vi "string parse mathematica list assosiated array -- V2.vi"(6 "pattern":string="^[\\t \\r \\n \\s \\, ]*\\\"(.+?)\\\"[\\t \\r \\n \\s]*\\-\\>[\\t \\r \\n \\s]*\\<\\|([^\\|]+)\\|\\>", 7 "action":T2=enum."parse string", 8 "array of inds":dbl[](array[numeric]), 9 "array of IDs":string[](array[string]), 10 "Map IN":map{string, map{T1, dbl}}(c390), 11 "string IN":string="\"014_042324\" ->   <|  \n\"T\"->  0.50  , \n\"θ\"-> 50 , \n\"vproj\" ->  0.3,\n\"B\" -> 60 ,\n\"plain\" -> \"bc\"\n  |>   , \n  \n\"012_042324\" ->   <|  \n\"T\"->  0.50  , \n\"θ\"-> 70  , \n\"vproj\" -> 0.5,\n\"plain\" -> \"bc\"\n  |>   ,  \n  \n  \n  ") -> (0 "items actually found":T1[](array[typedef])=[enum."T (K)", enum."B (T)", enum."θ (deg)"], 1 "actually found Map OUT":map{string, map{T1, dbl}}(c390)={"012_042324"={enum."T (K)"=0.5, enum."B (T)"=0.0, enum."θ (deg)"=70.0}, "014_042324"={enum."T (K)"=0.5, enum."B (T)"=60.0, enum."θ (deg)"=50.0}}, 2 "all keys Map OUT":map{string, map{T1, dbl}}(c390)={"012_042324"={enum."ζ"=0.0, enum."τ1"=0.0, enum."τS"=0.0, enum."τN"=0.0, enum."τC"=0.0, enum."κ0"=0.0, enum."m1"=0.0, enum."m2"=0.0, enum."m3"=0.0, enum."T (K)"=0.5, enum."B (T)"=0.0, enum."θ (deg)"=70.0, enum."Re(offset)"=0.0, enum."Im(offset)"=0.0, enum."στ1"=0.0, enum."στS"=0.0, enum."στN"=0.0, enum."τ11"=0.0, enum."τ12"=0.0, enum."τ22"=0.0, enum."τN1"=0.0, enum."τN2"=0.0, enum."σηlogτ1"=0.0, enum."σηlogτS"=0.0, enum."σηlogτN"=0.0, enum."σlogτ1"=0.0, enum."σlogτS"=0.0, enum."σlogτN"=0.0, enum."σητ1"=0.0, enum."σητS"=0.0, enum."σητN"=0.0, enum."noiseT"=0.0, enum."plain"=0.0, enum."vproj"=0.0}, "014_042324"={enum."ζ"=0.0, enum."τ1"=0.0, enum."τS"=0.0, enum."τN"=0.0, enum."τC"=0.0, enum."κ0"=0.0, enum."m1"=0.0, enum."m2"=0.0, enum."m3"=0.0, enum."T (K)"=0.5, enum."B (T)"=60.0, enum."θ (deg)"=50.0, enum."Re(offset)"=0.0, enum."Im(offset)"=0.0, enum."στ1"=0.0, enum."στS"=0.0, enum."στN"=0.0, enum."τ11"=0.0, enum."τ12"=0.0, enum."τ22"=0.0, enum."τN1"=0.0, enum."τN2"=0.0, enum."σηlogτ1"=0.0, enum."σηlogτS"=0.0, enum."σηlogτN"=0.0, enum."σlogτ1"=0.0, enum."σlogτS"=0.0, enum."σlogτN"=0.0, enum."σητ1"=0.0, enum."σητS"=0.0, enum."σητN"=0.0, enum."noiseT"=0.0, enum."plain"=0.0, enum."vproj"=0.0}}, 3 "string out":string="\"014_042324\" ->   <|  \n\"T\"->  0.50  , \n\"θ\"-> 50 , \n\"vproj\" = 0.3,\n\"B\" -> 60 ,\n\"plain\" -> \"bc\"\n  |>   , \n  \n\"012_042324\" ->   <|  \n\"T\"->  0.50  , \n\"θ\"-> 70  , \n\"vproj\" = 0.5,\n\"plain\" -> \"bc\"\n  |>   ,  \n  \n  \n  ")   [LabVIEW 2021]
uses:
  3-lorentzian-heat-response action.ctl
  3-lorentzian-parameters.ctl
  mathematica string map action.ctl
  3-lorentzian-heat-response -- V4.vi/142dd4c5-f9ed-c64b-bc14-a88e3e2c450a.vi
  <vilib>/Analysis/polynomials.llb/Polynomial Roots.vi
  <vilib>/Analysis/polynomials.llb/Polynomial Roots (DBL).vi
  <vilib>/Comparison/Less/Less Functor/Less Functor.lvclass
  <vilib>/regexp/Match Regular Expression.xnode
panel:
  out "after match":string
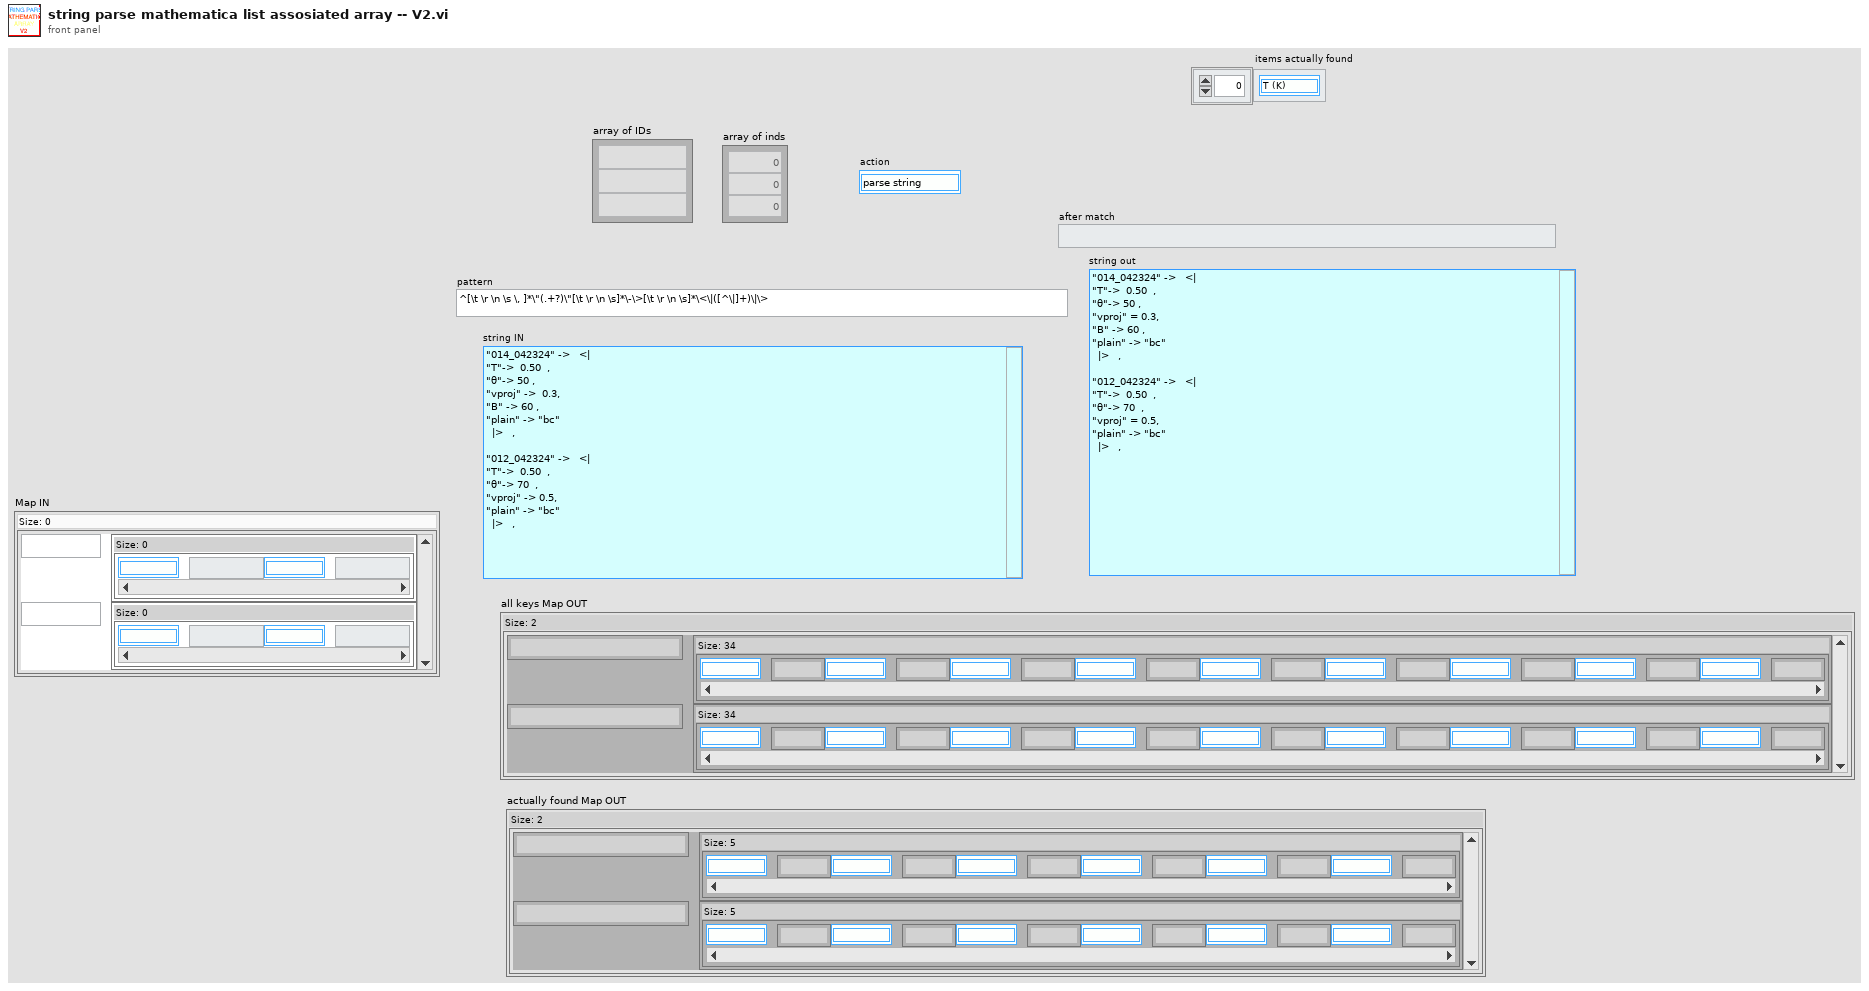
[diagram p1: front panel]
types:
  T1 = typedef "3-lorentzian-parameters.ctl" = enum16{"ζ", "τ1", "τS", "τN", "τC", "κ0", "m1", "m2", "m3", "T (K)", "B (T)", "θ (deg)", "side (S|R)", "set of (B|T)", "Re(offset)", "Im(offset)", "στ1", "στ1-", "στ1+", "στS", "στS-", "στS+", "στN", "στN-", "στN+", "τ11", "τ12", "τ21", "τ22", "τN1", "τN2", "σηlogτ1", "σηlogτS", "σηlogτN", "σlogτ1", "σlogτS", "σlogτN", "σητ1", "σητS", "σητN", "noiseT", "plain", "vproj"}
  T2 = typedef "3-lorentzian-heat-response action.ctl" = enum16{"calc R", "create string", "calc m1m2m3", "dζ", "dT1", "dτS", "dτN", "dτC", "d-all", "dκ0", "T(K)", "m1", "m2", "m3", "parse string", "θ (deg)", "B (T)", "onlygrads", "newton", "create emty string", "simple2nd", "calc R2", "ScalarProd", "ScalarProd-diff", "nothing", "ScalarProd-eta", "tolog", "ignore", "three2nd", "eta-errors"}
  T3 = typedef "mathematica string map action.ctl" = enum16{"create string", "calc m1m2m3", "parse string"}
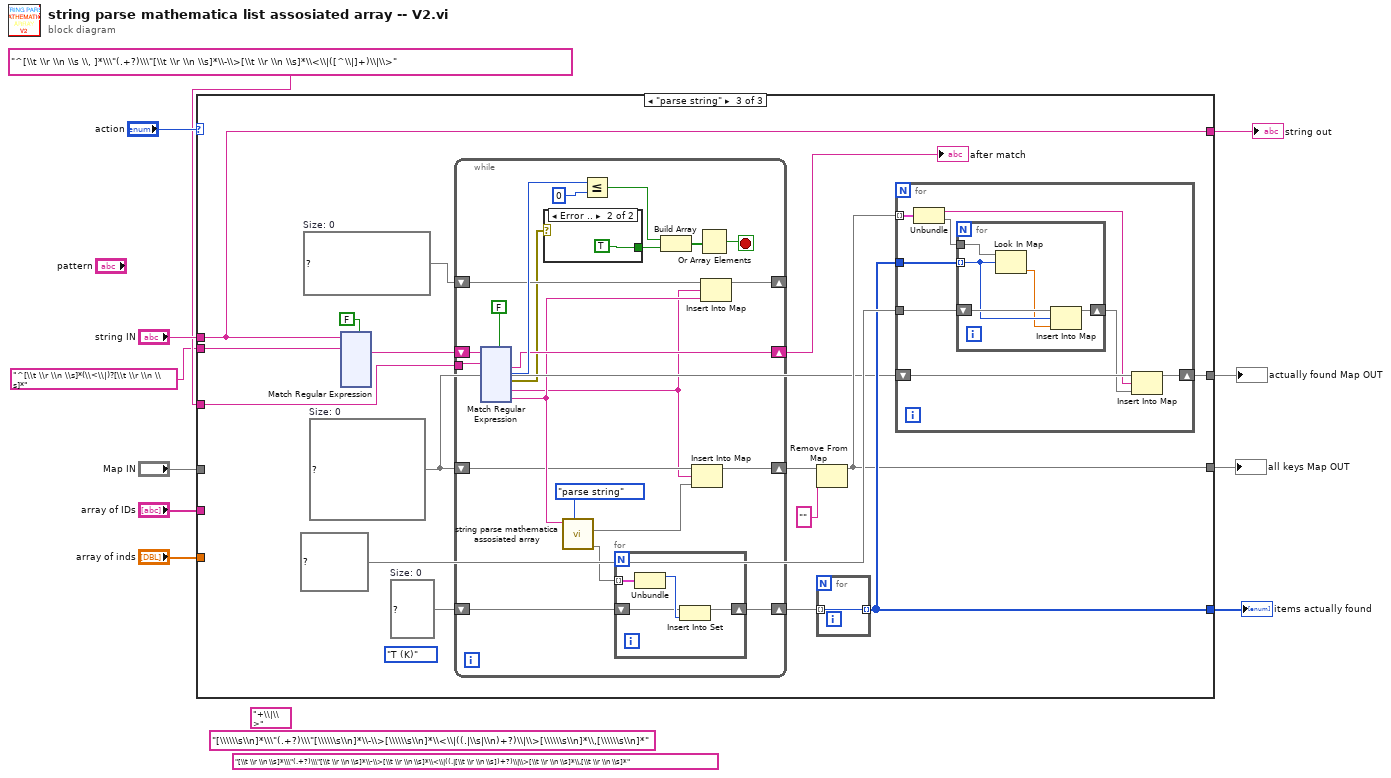
[diagram p0: block diagram]
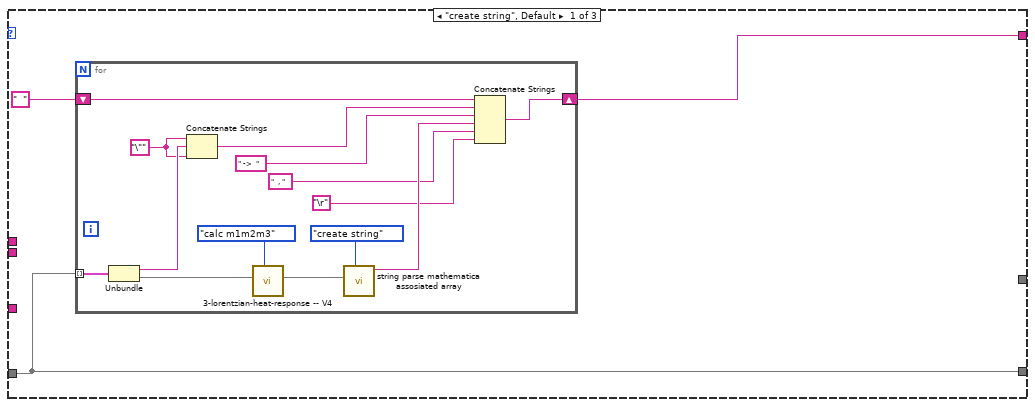
[diagram p2: hidden frame]
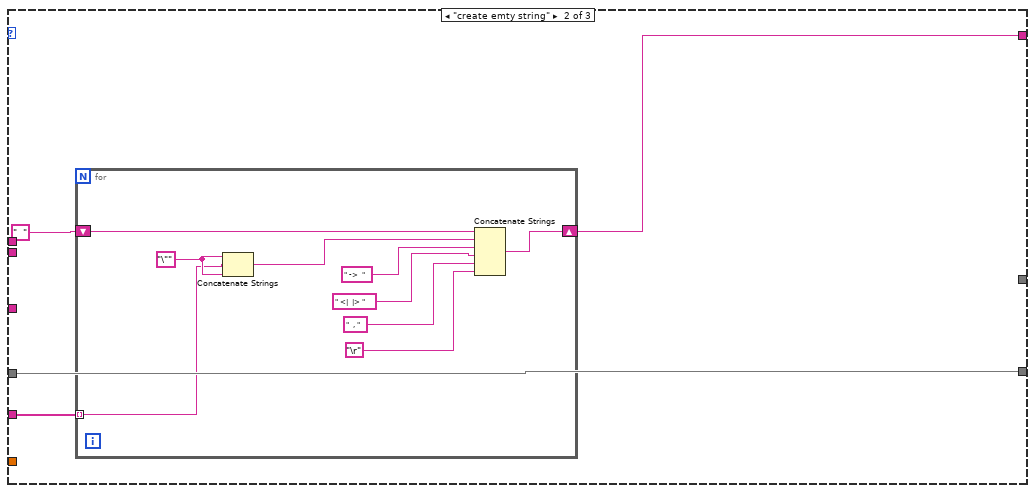
[diagram p3: hidden frame]
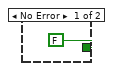
[diagram p4: hidden frame]
diagram:
  (unwired) "+\\|\\>" ("format string")
  (unwired) "[\\t \\r \\n \\s]*\\\"(.+?)\\\"[\\t \\r \\n \\s]*\\-\\>[\\t \\r \\n \\s]*\\<\\|((.|[\\t \\r \\n \\s])+?)\\|\\>[\\t \\r \\n \\s]*\\,[\\t \\r \\n \\s]*" ("pattern")
  (unwired) "[\\\\\\s\\n]*\\\"(.+?)\\\"[\\\\\\s\\n]*\\-\\>[\\\\\\s\\n]*\\<\\|((.|\\s|\\n)+?)\\|\\>[\\\\\\s\\n]*\\,[\\\\\\s\\n]*" ("pattern")
  n1 = case shown="\"parse string\"" "action" {
    tunnel: "string IN" -> [_ _ w53]
    tunnel: [w12 w30 w45] -> w6
    tunnel: "Map IN" -> [w12 w30 _]
    tunnel: [w14 w32 w53] -> w8
    tunnel: "array of inds" -> [_ _ _]
    tunnel: "array of IDs" -> [_ w29 _]
    tunnel: "^[\\t \\r \\n \\s \\, ]*\\\"(.+?)\\\"[\\t \\r \\n \\s]*\\-\\>[\\t \\r \\n \\s]*\\<\\|([^\\|]+)\\|\\>" ("pattern") -> [_ _ w49]
    tunnel: [_ _ w46] -> w3
    tunnel: [_ _ w44] -> w2
    tunnel: "^[\\t \\r \\n \\s]*(\\<\\|)?[\\t \\r \\n \\s]*" ("format string") -> [_ _ w42]
    frame "create string", Default {
      n2 = for {
        tunnel: w12 -> [w28] mode=indexing
        shift-right: [w22] -> w14
        shift-left: "  " ("all string") -> [w23]
        w15 = "\"" ("all string")
        n3 = Unbundle(w28) -> ("after match 3"=w17:string, "Map"=w20:map{T1, dbl})
        n4 = Concatenate Strings(w15, w17, w15) -> (w16:string)
        n5 = call "3-lorentzian-heat-response -- V4.vi"("action"=3-lorentzian-heat-response_action."calc m1m2m3", "Map IN"=w20) -> ("Map OUT"=w18:map{T1, dbl})  [unwired: 7 in, 2 out]
        n6 = call "string parse mathematica assosiated array.vi"("action"=mathematica_string_map_action."create string" ("derivative"), "map IN"=w18) -> ("String OUT"=w26:string)  [unwired: 7 in, 2 out]
        n7 = Concatenate Strings(w23, w16, " ->  " ("all string"), w26, "  , " ("all string"), "\r") -> (w22:string)
      }
    }
    frame "create emty string" {
      n8 = for {
        shift-right: [w38] -> w32
        shift-left: "  " ("all string") -> [w39]
        tunnel: w29 -> [w34] mode=indexing
        w35 = "\"" ("all string")
        n9 = Concatenate Strings(w35, w34, w35) -> (w33:string)
        n10 = Concatenate Strings(w39, w33, " ->  " ("all string"), " <|  |> " ("all string"), "  , " ("all string"), "\r") -> (w38:string)
      }
    }
    frame "parse string" {
      (unwired) 3-lorentzian-parameters."T (K)" ("Plost: sweep window")
      w50 = set{T1} {}  # Size: 0
      w43 = map{string, map{T1, dbl}} {}  # Size: 0
      w56 = map{string, string} {}  # Size: 0
      n11 = xnode "Match Regular Expression"("input string"=w53, "regular expression"=w42, "multiline? (F)"=FALSE) -> ("after match"=w57:string)  [unwired: 3 in, 6 out]
      n12 = while {
        shift-right: [w90] -> w55
        shift-left: w57 -> [w93]
        shift-right: [w88] -> _
        shift-left: w56 -> [w89]
        shift-right: [w83] -> w54
        shift-left: w43 -> [w85]
        shift-right: [w73] -> w48
        shift-left: w50 -> [w74]
        tunnel: w49 -> [w75]
        stop <- w79 stop-if-true
        n13 = xnode "Match Regular Expression"("input string"=w93, "regular expression"=w75, "multiline? (F)"=FALSE) -> ("after match"=w90:string, "offset past match"=w92:i32, "error out"=w80:errorcluster, "submatch 1"=w76:string, "submatch 2"=w86:string)  [unwired: 3 in, 2 out]
        n14 = case shown="Error .." w80 {
          tunnel: [FALSE TRUE] -> w77
          frame No Error {
          }
          frame Error {
          }
        }
        n15 = call "string parse mathematica assosiated array.vi"("action"=mathematica_string_map_action."parse string" ("derivative"), "String in"=w86) -> ("actually found"=w72:map{T1, string}, "Map OUT"=w84:map{T1, dbl})  [unwired: 7 in, 1 out]
        n16 = Less Or Equal?(x=w92, y=0) -> (x <= y?=w81:bool)
        n17 = for {
          shift-right: [w95] -> w73
          shift-left: w74 -> [w96]
          tunnel: w72 -> [w94] mode=indexing
          n18 = Unbundle(w94) -> ("Plost: sweep window"=w97:T1)  [unwired: 1 out]
          n19 = Insert Into Set(10:w97, 11:w96) -> (3:w95:set{T1})  [unwired: 1 out]
        }
        n20 = Build Array(w81, w77) -> (w78:bool[])
        n21 = Insert Into Map(map in=w85, key=w76, value=w84) -> (map out=w83:map{string, map{T1, dbl}})  [unwired: 2 out]
        n22 = Or Array Elements(Boolean array=w78) -> (logical OR=w79:bool)
        n23 = Insert Into Map(map in=w89, key=w76, value=w86) -> (map out=w88:map{string, string})  [unwired: 2 out]
      }
      "after match" <- w55
      n24 = Remove From Map(10:"" ("format string"), 11:w54) -> (3:w45:map{string, map{T1, dbl}})  [unwired: 2 out]
      n25 = for {
        tunnel: w48 -> [w71] mode=indexing
        tunnel: [w71] -> w46 mode=indexing
      }
      n26 = for {
        tunnel: w45 -> [w65] mode=indexing
        shift-right: [w60] -> w44
        shift-left: w43 -> [w61]
        tunnel: w46 -> [w64]
        tunnel: map{T1, dbl} {} ("Map") -> [w62]
        n27 = Unbundle(w65) -> ("format string"=w59:string, w63:map{T1, dbl})
        n28 = for {
          tunnel: w64 -> [w69] mode=indexing
          shift-right: [w67] -> w58
          shift-left: w62 -> [w70]
          tunnel: w63 -> [w66]
          n29 = Look In Map(map=w66, key=w69) -> (value=w68:dbl)  [unwired: 1 in, 1 out]
          n30 = Insert Into Map(map in=w70, key=w69, value=w68) -> (map out=w67:map{T1, dbl})  [unwired: 2 out]
        }
        n31 = Insert Into Map(map in=w61, key=w59, value=w58) -> (map out=w60:map{string, map{T1, dbl}})  [unwired: 2 out]
      }
    }
  }
  "string out" <- w8
  "all keys Map OUT" <- w6
  "items actually found" <- w3
  "actually found Map OUT" <- w2
